vi "Input Channel Page.vi"(8 "error in":errorcluster, 11 "Node Ptr":T1 format="%.0x") -> (0 "error out":errorcluster)   [LabVIEW 2026]
uses:
  <vilib>/NI VeriStand/Custom Device API/Custom Device Item Ref.ctl
  C:/Program Files/National Instruments/VeriStand 2026/NationalInstruments.VeriStand.Controls.dll
  Program Files/National Instruments/VeriStand 2026/NationalInstruments.VeriStand.Controls.dll
  <vilib>/NI VeriStand/Custom Device API/Custom Device API.lvlib
  Template System Explorer.lvlib
panel:
  in  "PagePropertyEditor":refnum<k24>(container)
  out "Channel":string[][](table) caption="Channel Settings"
  in  "Default Value":dbl
  in  "General Header":cluster{"Section Name":string}={"Section Name"="Custom Device Channel Specification"}
  in  "Description":string
  in  "Name":string
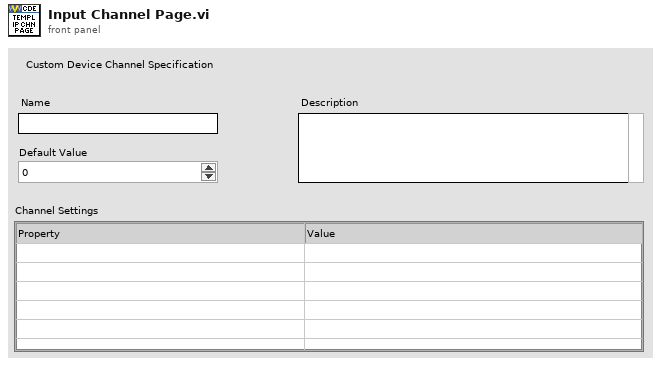
[diagram p1: front panel]
types:
  T1 = typedef "Custom Device API.lvlib/Custom Device Item Ref.ctl" = u64
  T2 = typedef "Custom Device API.lvlib/Custom Device Item Info.ctl" = cluster{"Name":string, "Is Channel":bool, "GUID":string, "Is Waveform":bool}
  T3 = typedef "Custom Device API.lvlib/Custom Device Commands.ctl" = enum16{"Default", "Item renamed", "Shutdown", "Dynamic button pressed"}
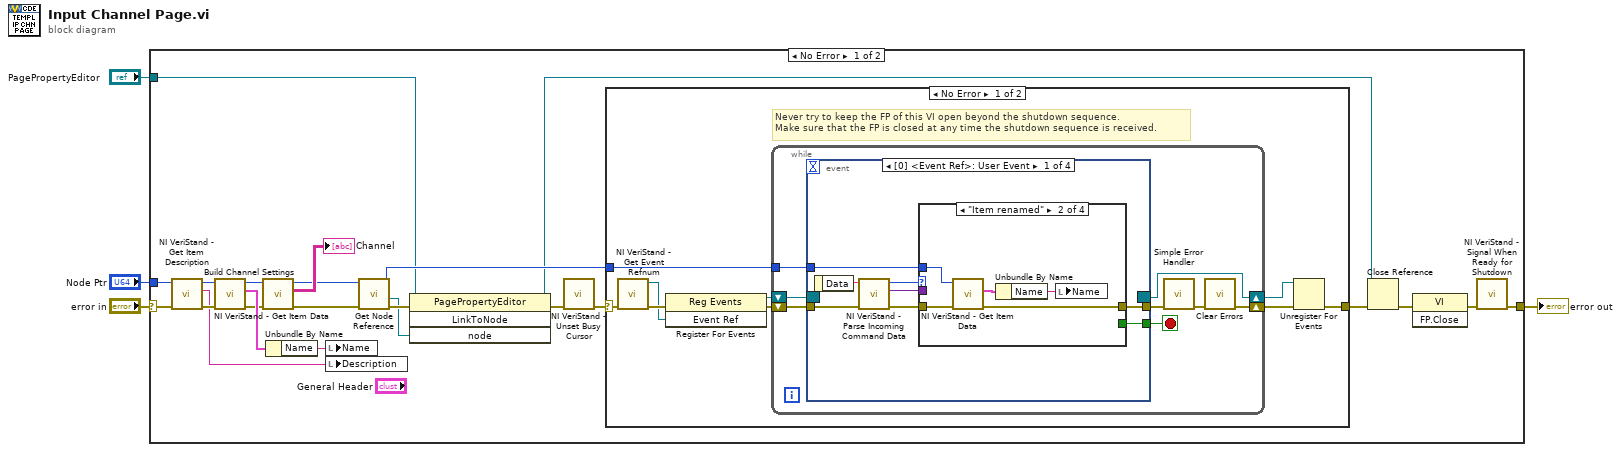
[diagram p0: block diagram]
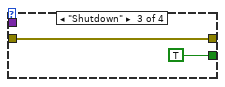
[diagram p3: hidden frame]
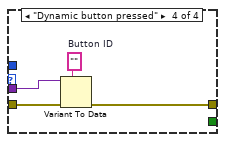
[diagram p4: hidden frame]
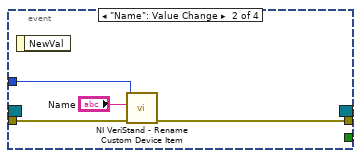
[diagram p5: hidden frame]
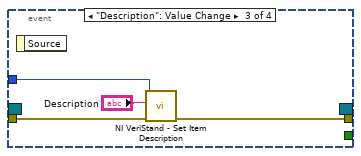
[diagram p6: hidden frame]
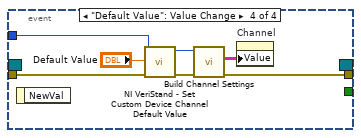
[diagram p7: hidden frame]
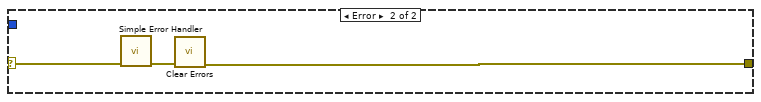
[diagram p8: hidden frame]
diagram:
  n1 = case shown="No Error" "error in" {
    selector: "error in" -> [w22 w83]
    tunnel: [w27 w83] -> w2
    tunnel: "Node Ptr" -> [w21 _]
    tunnel: "PagePropertyEditor" -> [w20 _]
    frame No Error {
      n2 = call <vilib>:"NI VeriStand - Get Item Description.vi"("error in (no error)"=w22, "Item Ref in"=w21) -> ("error out"=w19:errorcluster, "Description"=w15:string, "Item Ref out"=w18:T1)  [unwired: 7 out]
      n3 = call <vilib>:"NI VeriStand - Get Item Data.vi"("error in (no error)"=w19, "Item Ref in"=w18) -> ("error out"=w14:errorcluster, "Item Info"=w17:T2, "Item Ref out"=w13:T1)  [unwired: 7 out]
      n4 = call "Build Channel Settings.vi"("error in"=w14, "Node Ptr"=w13) -> ("error out"=w10:errorcluster, "Channel Settings Table"=→"Channel":string[][], "Node Ptr out"=w9:T1)  [unwired: 7 in]
      n5 = Unbundle By Name(w17) -> ("Name"=w16:string)
      n6 = local write "Name"(w16) -> ()
      n7 = local write "Description"(w15) -> ()
      n8 = call "Get Node Reference.vi"("error in"=w10, "Node Ptr"=w9) -> ("error out"=w11:errorcluster, "Base Node"=w8:refnum<k24>, "Node Ptr"=w24:T1)  [unwired: 6 in, 1 out]
      n9 = invoke class="PagePropertyEditor" method="LinkToNode"(reference=w20, error in=w11, "node"=w8) -> (reference out=w5:refnum<k24>, error out=w23:errorcluster)  [unwired: 1 in, 2 out]
      n10 = call <vilib>:"NI VeriStand - Unset Busy Cursor.vi"("error in (no error)"=w23) -> ("error out"=w25:errorcluster)  [unwired: 10 out]
      n11 = case shown="No Error" w25 {
        selector: w25 -> [w32 w82]
        tunnel: [w34 w80] -> w7
        tunnel: w24 -> [w28 _]
        frame No Error {
          # "Never try to keep the FP of this VI open beyond the shutdown sequence.\nMake sure that the FP is closed at any time the shutdown sequence is received."
          n12 = call <vilib>:"NI VeriStand - Get Event Refnum.vi"("error in (no error)"=w32) -> ("error out"=w36:errorcluster, "Event Ref"=w30:refnum<user-event>)  [unwired: 9 out]
          n13 = register-events(error in=w36, w30) -> (reference out=w29:refnum<event-registration>, error out=w33:errorcluster)  [unwired: 1 in]
          n14 = while {
            tunnel: w28 -> [w37]
            shift-right: [w41] -> w35
            shift-left: w33 -> [w44]
            shift-right: [w40] -> w31
            shift-left: w29 -> [w39]
            stop <- w38 stop-if-true
            n15 = event shown="[0] <Event Ref>: User Event" {
              selector: w39 -> [_ _ _ _]
              dyn-events: [_ _ _ _] -> w40
              timeout: _ -> [_ _ _ _]
              tunnel: w44 -> [w52 w68 w72 w77]
              tunnel: [w47 _ _ _] -> w38
              tunnel: [w50 w67 w71 w79] -> w43
              tunnel: w37 -> [w46 w66 w70 w73]
              event User Event {
                n16 = event-data() -> ("Data"=w49:string)  [unwired: 1 out]
                n17 = call <vilib>:"NI VeriStand - Parse Incoming Command Data.vi"("error in (no error)"=w52, "Incoming data"=w49) -> ("error out"=w51:errorcluster, "Outgoing data"=w45:variant, "Action"=w48:T3)  [unwired: 7 out]
                n18 = case shown="\"Item renamed\"" w48 {
                  tunnel: w51 -> [w53 w58 w60 w64]
                  tunnel: [_ _ TRUE _] -> w47
                  tunnel: [w53 w57 w60 w63] -> w50
                  tunnel: w46 -> [_ w56 _ _]
                  tunnel: w45 -> [_ _ _ w62]
                  frame "Default", Default {
                  }
                  frame "Item renamed" {
                    n19 = call <vilib>:"NI VeriStand - Get Item Data.vi"("error in (no error)"=w58, "Item Ref in"=w56) -> ("error out"=w57:errorcluster, "Item Info"=w55:T2)  [unwired: 8 out]
                    n20 = Unbundle By Name(w55) -> ("Name"=w54:string)
                    n21 = local write "Name"(w54) -> ()
                  }
                  frame "Shutdown" {
                  }
                  frame "Dynamic button pressed" {
                    w61 = ""  # Button ID
                    n22 = Variant To Data(error in=w64, type=w61, Variant=w62) -> (error out=w63:errorcluster)  [unwired: 1 out]
                  }
                }
              }
              event "Name": Value Change {
                n23 = event-data() -> ()  [unwired: 2 out]
                n24 = call <vilib>:"NI VeriStand - Rename Custom Device Item.vi"("error in (no error)"=w68, "New Name"="Name", "Item Ref in"=w66) -> ("error out"=w67:errorcluster)  [unwired: 1 in, 7 out]
              }
              event "Description": Value Change {
                n25 = event-data() -> ()  [unwired: 2 out]
                n26 = call <vilib>:"NI VeriStand - Set Item Description.vi"("error in (no error)"=w72, "Description"="Description", "Item Ref in"=w70) -> ("error out"=w71:errorcluster)  [unwired: 8 out]
              }
              event "Default Value": Value Change {
                n27 = event-data() -> ()  [unwired: 2 out]
                n28 = call <vilib>:"NI VeriStand - Set Custom Device Channel Default Value.vi"("error in (no error)"=w77, "Default Value"="Default Value", "Channel Ref in"=w73) -> ("error out"=w76:errorcluster, "Channel Ref out"=w74:T1)  [unwired: 7 in]
                n29 = call "Build Channel Settings.vi"("error in"=w76, "Node Ptr"=w74) -> ("error out"=w79:errorcluster, "Channel Settings Table"=w78:string[][])  [unwired: 7 in, 1 out]
                n30 = property on="Channel" class="Tbl (strict)"("Value"=w78) -> ()  [unwired: 2 in, 2 out]
              }
            }
            n31 = call <vilib>:"Simple Error Handler.vi"("error in (no error)"=w43) -> ("error out"=w42:errorcluster)  [unwired: 1 in, 7 out]
            n32 = call <vilib>:"Clear Errors.vi"("error in (no error)"=w42) -> ("error out"=w41:errorcluster)  [unwired: 1 in, 5 out]
          }
          n33 = Unregister For Events(event registration refnum=w31, error in=w35) -> (error out=w34:errorcluster)
        }
        frame Error {
          n34 = call <vilib>:"Simple Error Handler.vi"("error in (no error)"=w82) -> ("error out"=w81:errorcluster)  [unwired: 1 in, 7 out]
          n35 = call <vilib>:"Clear Errors.vi"("error in (no error)"=w81) -> ("error out"=w80:errorcluster)  [unwired: 1 in, 5 out]
        }
      }
      n36 = Close Reference(reference=w5, error in (no error)=w7) -> (error out=w6:errorcluster)
      n37 = invoke class="VI" method="FP.Close"(error in=w6) -> (error out=w26:errorcluster)  [unwired: 2 in, 2 out]
      n38 = call <vilib>:"NI VeriStand - Signal When Ready for Shutdown.vi"("error in (no error)"=w26) -> ("error out"=w27:errorcluster)  [unwired: 10 out]
    }
    frame Error {
    }
  }
  "error out" <- w2
